vi "Vision Analisis.vi"(8 "error in":errorcluster, 9 "Linha 2":string, 10 "Linha 1":string, 11 "Image Case":T2) -> (0 "error out":errorcluster, 1 "Gabarito":string, 2 "Passed?":bool, 3 "String (OCR/OCV 1)":string, 4 "Image Out":T1(plugin-control))   [LabVIEW 2016, in "MVP02 Custom Device.lvlib"]
uses:
  MVP02 Custom Device.lvlib
  Vision Case.ctl
  <vilib>/vision/Image Controls.llb/IMAQ Image.ctl
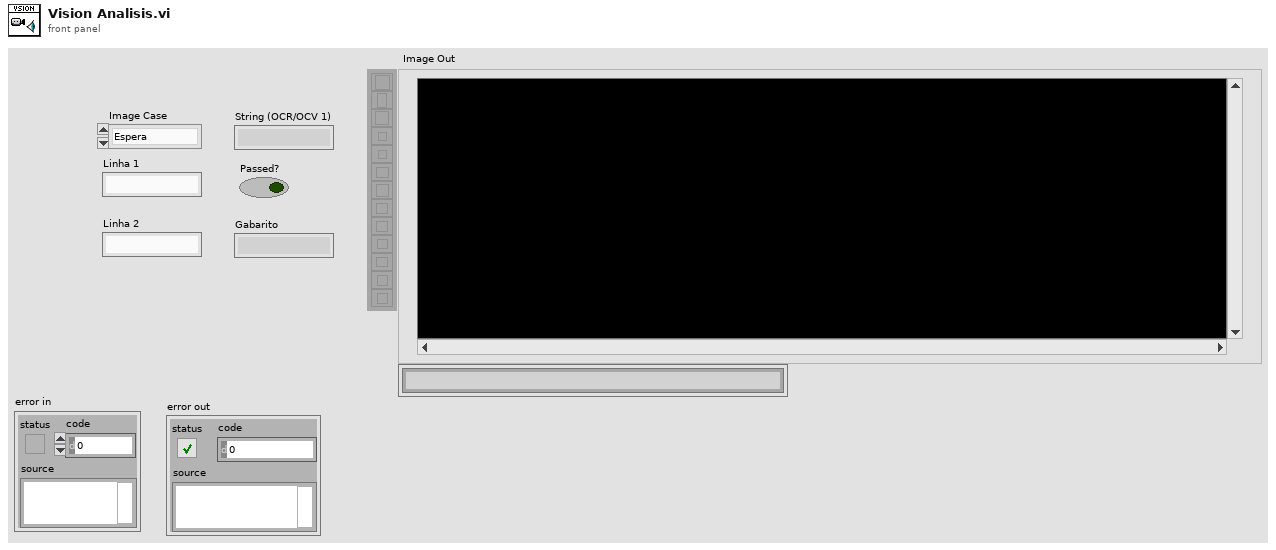
[diagram p1: front panel]
types:
  T1 = typedef "IMAQ Image.ctl" = refnum<image>
  T2 = typedef "Vision Case.ctl" = enum16{"Espera", "OCR", "OCR2", "Outros"}
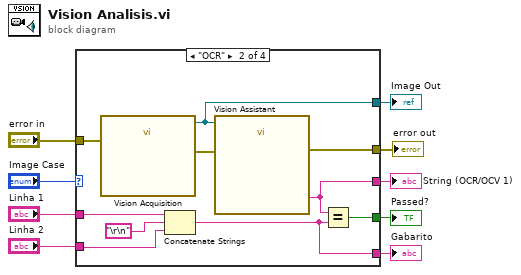
[diagram p0: block diagram]
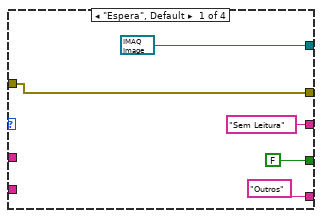
[diagram p2: hidden frame]
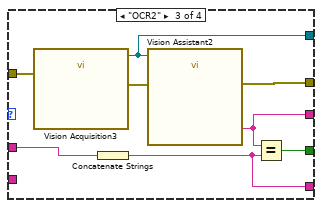
[diagram p3: hidden frame]
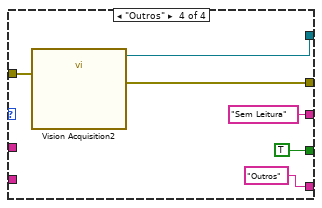
[diagram p4: hidden frame]
diagram:
  n1 = case shown="\"OCR\"" "Image Case" {
    tunnel: "Linha 1" -> [_ w23 w32 _]
    tunnel: "Linha 2" -> [_ w22 _ _]
    tunnel: [FALSE w16 w26 TRUE] -> w9
    tunnel: "error in" -> [w13 w21 w31 w35]
    tunnel: [w13 w19 w29 w34] -> w4
    tunnel: ["Sem Leitura" ("String (OCR/OCV 1)") w18 w28 "Sem Leitura" ("String (OCR/OCV 1)")] -> w3
    tunnel: ["Outros" w17 w27 "Outros"] -> w2
    tunnel: [T1 refnum ("Image Out") w15 w25 w33] -> w1
    frame "Espera", Default {
    }
    frame "OCR" {
      n2 = call "Vision Acquisition"("error in"=w21) -> ("Image Out"=w15:T1, "error out"=w20:errorcluster)  [unwired: 25 in]
      n3 = Concatenate Strings(w23, "\r\n", w22) -> (w17:string)
      n4 = call "Vision Assistant"("Image In"=w15, "error in"=w20) -> ("String (OCR/OCV 1)"=w18:string, "error out"=w19:errorcluster)  [unwired: 22 in, 2 out]
      n5 = Equal?(x=w18, y=w17) -> (x = y?=w16:bool)
    }
    frame "OCR2" {
      n6 = call "Vision Acquisition3"("error in"=w31) -> ("Image Out"=w25:T1, "error out"=w30:errorcluster)  [unwired: 25 in]
      n7 = Concatenate Strings(w32) -> (w27:string)
      n8 = call "Vision Assistant2"("Image In"=w25, "error in"=w30) -> ("String (OCR/OCV 1)"=w28:string, "error out"=w29:errorcluster)  [unwired: 23 in, 1 out]
      n9 = Equal?(x=w28, y=w27) -> (x = y?=w26:bool)
    }
    frame "Outros" {
      n10 = call "Vision Acquisition2"("error in"=w35) -> ("Image Out"=w33:T1, "error out"=w34:errorcluster)  [unwired: 25 in]
    }
  }
  "Passed?" <- w9
  "error out" <- w4
  "String (OCR/OCV 1)" <- w3
  "Gabarito" <- w2
  "Image Out" <- w1
